vi "Teleop.vi"(10 "Match Info":T1={"Autonomous Elapsed Seconds"=0.0, "TeleOp Elapsed Seconds"=0.0, "Disabled Elapsed Seconds"=0.0, "Visited Autonomous"=FALSE, "Visited TeleOp"=FALSE, "Visited Disabled"=FALSE, "Autonomous Settings"={"Autonomous Style"=enum."Independent", "VI Refnum"=refnum}}, 11 "Call Context":T2) -> ()   [LabVIEW 2017]
doc: "This VI is called for each enabled TeleOp packet received from the DS. It is typically used to read from joysticks and other inputs and update I/O or setpoints for timed control loops. It should complete and return within 20 milliseconds or risk missing DS packets."
uses:
  <vilib>/Rock Robotics/WPI/DriverStation/WPI_DriverStationDerivedRobotMode.ctl
  <vilib>/Rock Robotics/WPI/DriverStation/WPI_DriverStationMatch Info.ctl
  <vilib>/Rock Robotics/WPI/Utilities/WPI_GetSetVariantRefNum.vi
  <vilib>/Rock Robotics/Network Tables/NT Write Boolean Array.vi
  <vilib>/Rock Robotics/Network Tables/NT Write Numeric Array.vi
panel:
  in  "Climber Rate":dbl=0.8
  in  "Hook Arm Rate":dbl=0.8
  out "Lower Arm":bool
  out "Lift Arm":bool
  in  "Arm Rate":dbl=0.8
  in  "Turn Rate":dbl=0.5
  in  "Speed Rate":dbl=0.5
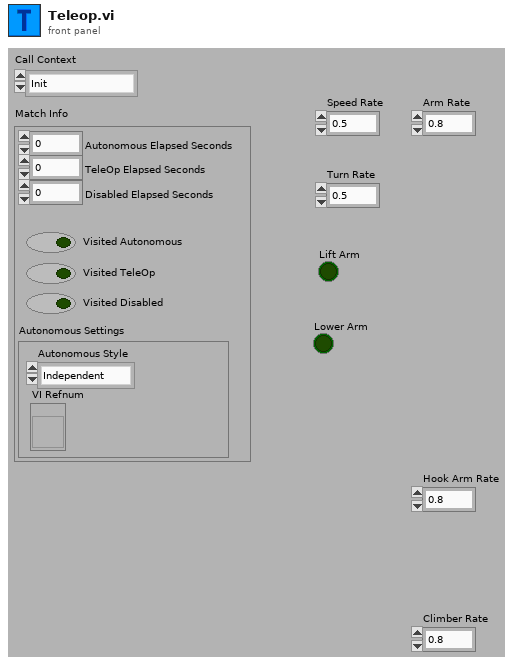
[diagram p1: front panel]
types:
  T1 = typedef "WPI_DriverStationMatch Info.ctl" = cluster{"Autonomous Elapsed Seconds":dbl, "TeleOp Elapsed Seconds":dbl, "Disabled Elapsed Seconds":dbl, "Visited Autonomous":bool, "Visited TeleOp":bool, "Visited Disabled":bool, "Autonomous Settings":cluster{"Autonomous Style":enum16{"Iterative", "Independent"}, "VI Refnum":refnum<vi>}}
  T2 = typedef "WPI_DriverStationDerivedRobotMode.ctl" = enum16{"Init", "Execute", "Stop"}
  T3 = typedef "WPI_JoystickDevRef.ctl" = cluster{"Device":T4}
  T4 = typedef "WPI_JoystickDeviceEnum.ctl" = enum16{"USB 0", "USB 1", "USB 2", "USB 3", "USB 4", "USB 5"}
  T5 = typedef "Command Status Info.ctl" = cluster{"Name":string, "Status":T6, "notifier out":T7}
  T6 = typedef "Completion Status.ctl" = enum16{"Successful", "Aborted", "Incomplete"}
  T7 = typedef "Completion Notifier.ctl" = refnum<notifier>
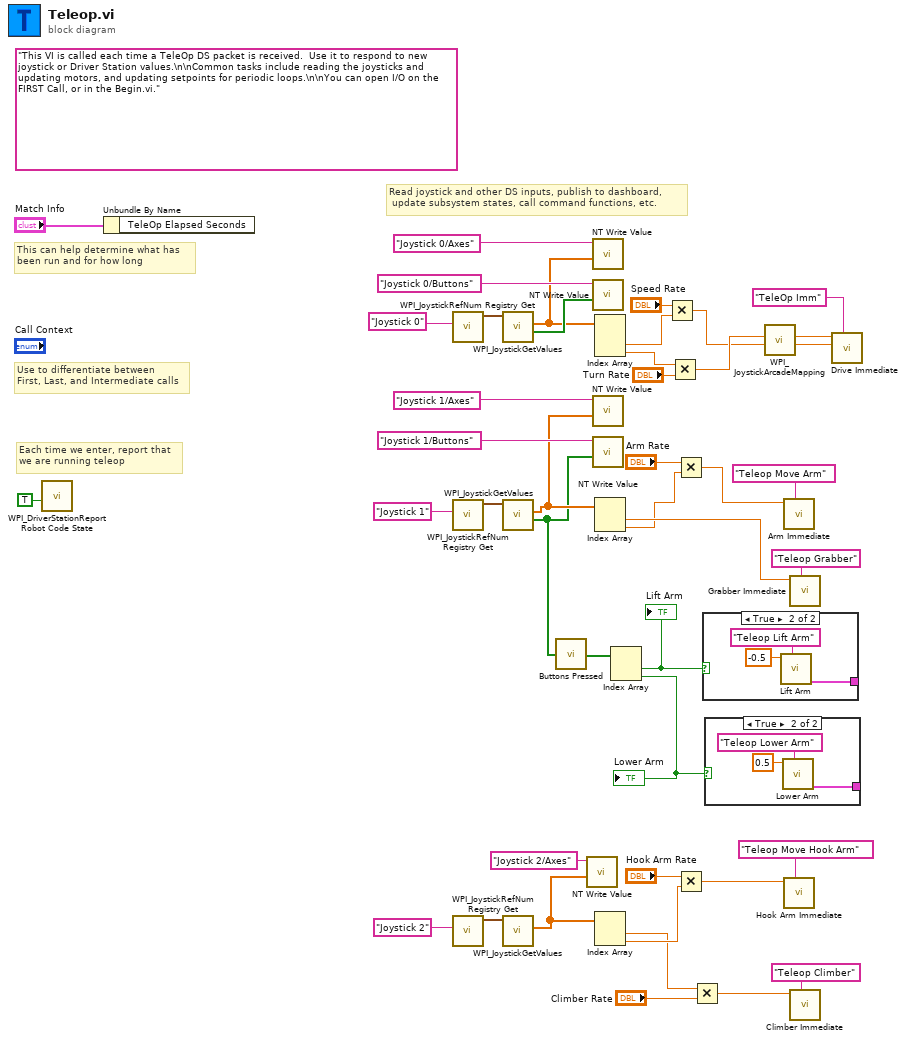
[diagram p0: block diagram]
diagram:
  (unwired) "This VI is called each time a TeleOp DS packet is received.  Use it to respond to new joystick or Driver Station values.\n\nCommon tasks include reading the joysticks and updating motors, and updating setpoints for periodic loops.\n\nYou can open I/O on the FIRST Call, or in the Begin.vi."
  # "Read joystick and other DS inputs, publish to dashboard,\n update subsystem states, call command functions, etc."
  # "Each time we enter, report that\nwe are running teleop"
  # "Use to differentiate between\nFirst, Last, and Intermediate calls"
  # "This can help determine what has\nbeen run and for how long"
  n1 = call <vilib>:"WPI_DriverStationReport Robot Code State.vi"("TeleOp"=TRUE ("Autonomous")) -> ()  [unwired: 10 in, 1 out]
  n2 = Unbundle By Name("Match Info") -> ()  [unwired: 1 out]
  n3 = call <vilib>:"WPI_JoystickRefNum Registry Get.vi"("refnum name"="Joystick 0") -> ("JoystickDevRef"=w41:T3)  [unwired: 1 in, 9 out]
  n4 = call <vilib>:"WPI_JoystickRefNum Registry Get.vi"("refnum name"="Joystick 1") -> ("JoystickDevRef"=w33:T3)  [unwired: 1 in, 9 out]
  n5 = call <vilib>:"WPI_JoystickRefNum Registry Get.vi"("refnum name"="Joystick 2") -> ("JoystickDevRef"=w3:T3)  [unwired: 1 in, 9 out]
  n6 = call <vilib>:"WPI_JoystickGetValues.vi"("JoystickDevRef"=w41) -> ("Buttons"=w36:bool[], "Axes"=w35:dbl[])  [unwired: 6 in, 3 out]
  n7 = call <vilib>:"WPI_JoystickGetValues.vi"("JoystickDevRef"=w33) -> ("Buttons"=w13:bool[], "Axes"=w14:dbl[])  [unwired: 6 in, 3 out]
  n8 = call <vilib>:"WPI_JoystickGetValues.vi"("JoystickDevRef"=w3) -> ("Axes"=w2:dbl[])  [unwired: 6 in, 4 out]
  n9 = call "Buttons Pressed.vi"("Button Values"=w13) -> ("Button Presses"=w19:bool[])
  n10 = call-poly <vilib>:"NT Write Value.vi"("Numeric Array"=w2, "Name"="Joystick 2/Axes") -> ()  [unwired: 9 in, 1 out]
  n11 = call-poly <vilib>:"NT Write Value.vi"("Numeric Array"=w35, "Name"="Joystick 0/Axes") -> ()  [unwired: 9 in, 1 out]
  n12 = call-poly <vilib>:"NT Write Value.vi"("Boolean Array"=w36, "Name"="Joystick 0/Buttons") -> ()  [unwired: 9 in, 1 out]
  n13 = call-poly <vilib>:"NT Write Value.vi"("Numeric Array"=w14, "Name"="Joystick 1/Axes") -> ()  [unwired: 9 in, 1 out]
  n14 = call-poly <vilib>:"NT Write Value.vi"("Boolean Array"=w13, "Name"="Joystick 1/Buttons") -> ()  [unwired: 9 in, 1 out]
  n15 = Index Array(array=w35) -> (element #2=w26:dbl, element #3=w28:dbl)  [unwired: 3 in, 1 out]
  n16 = Index Array(array=w14) -> (element #1=w30:dbl, element #2=w21:dbl)  [unwired: 2 in]
  n17 = Index Array(array=w2) -> (element #1=w6:dbl, element #2=w11:dbl)  [unwired: 2 in]
  n18 = Index Array(array=w19) -> (element #1=w18:bool, element #2=w17:bool)  [unwired: 2 in]
  "Lift Arm" <- w18
  "Lower Arm" <- w17
  n19 = Multiply(x="Speed Rate", y=w26) -> (x*y=w25:dbl)
  n20 = Multiply(x=w28, y="Turn Rate") -> (x*y=w27:dbl)
  n21 = Multiply(x="Arm Rate", y=w21) -> (x*y=w20:dbl)
  n22 = Multiply(x="Hook Arm Rate", y=w11) -> (x*y=w12:dbl)
  n23 = Multiply(x=w6, y="Climber Rate") -> (x*y=w5:dbl)
  n24 = case shown="True" w18 {
    tunnel: [_ w46] -> _
    frame False {
    }
    frame True {
      n25 = call "Lift Arm.vi"("Description"="Teleop Lift Arm", "Setpoint"=-0.5) -> ("Command Info Out"=w46:T5)  [unwired: 9 in]
    }
  }
  n26 = case shown="True" w17 {
    tunnel: [_ w49] -> _
    frame False {
    }
    frame True {
      n27 = call "Lower Arm.vi"("Description"="Teleop Lower Arm", "Setpoint"=0.5) -> ("Command Info Out"=w49:T5)  [unwired: 9 in]
    }
  }
  n28 = call <vilib>:"WPI_JoystickArcadeMapping.vi"("Y axis value"=w25, "X axis value"=w27) -> ("Right Motor Value"=w38:dbl, "Left Motor Value"=w39:dbl)  [unwired: 8 in]
  n29 = call "Arm Immediate.vi"("Description"="Teleop Move Arm", "Setpoint"=w20) -> ()  [unwired: 9 in, 1 out]
  n30 = call "Hook Arm Immediate.vi"("Description"="Teleop Move Hook Arm", "Setpoint"=w12) -> ()  [unwired: 9 in, 1 out]
  n31 = call "Grabber Immediate.vi"("Description"="Teleop Grabber", "Setpoint"=w30) -> ()  [unwired: 9 in, 1 out]
  n32 = call "Climber Immediate.vi"("Description"="Teleop Climber", "Setpoint"=w5) -> ()  [unwired: 9 in, 1 out]
  n33 = call "Drive Immediate.vi"("Description"="TeleOp Imm", "Right Setpoint"=w38, "Left Setpoint"=w39) -> ()  [unwired: 8 in, 1 out]
